vi "Unevenly Sampled Signal Spectrum.vi"(0 "XTime":dbl[](array[numeric]), 1 "X":dbl[](array[numeric])) -> (2 "Power Spectrum FFT {X} Frequency":dbl[](array[numeric]), 3 "Power Spectrum FFT {X}":dbl[](array[numeric]), 4 "error":i32)   [LabVIEW 2024, in "NI_Gmath.lvlib"]
doc: "<p>Calculates the power spectrum of a signal that is unevenly spaced in time.</p>"
uses:
  NI_Gmath.lvlib
  Real Dot Product.vi
  NI_AALBase.lvlib
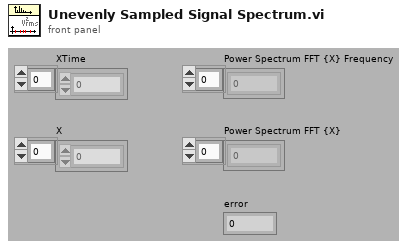
[diagram p1: front panel]
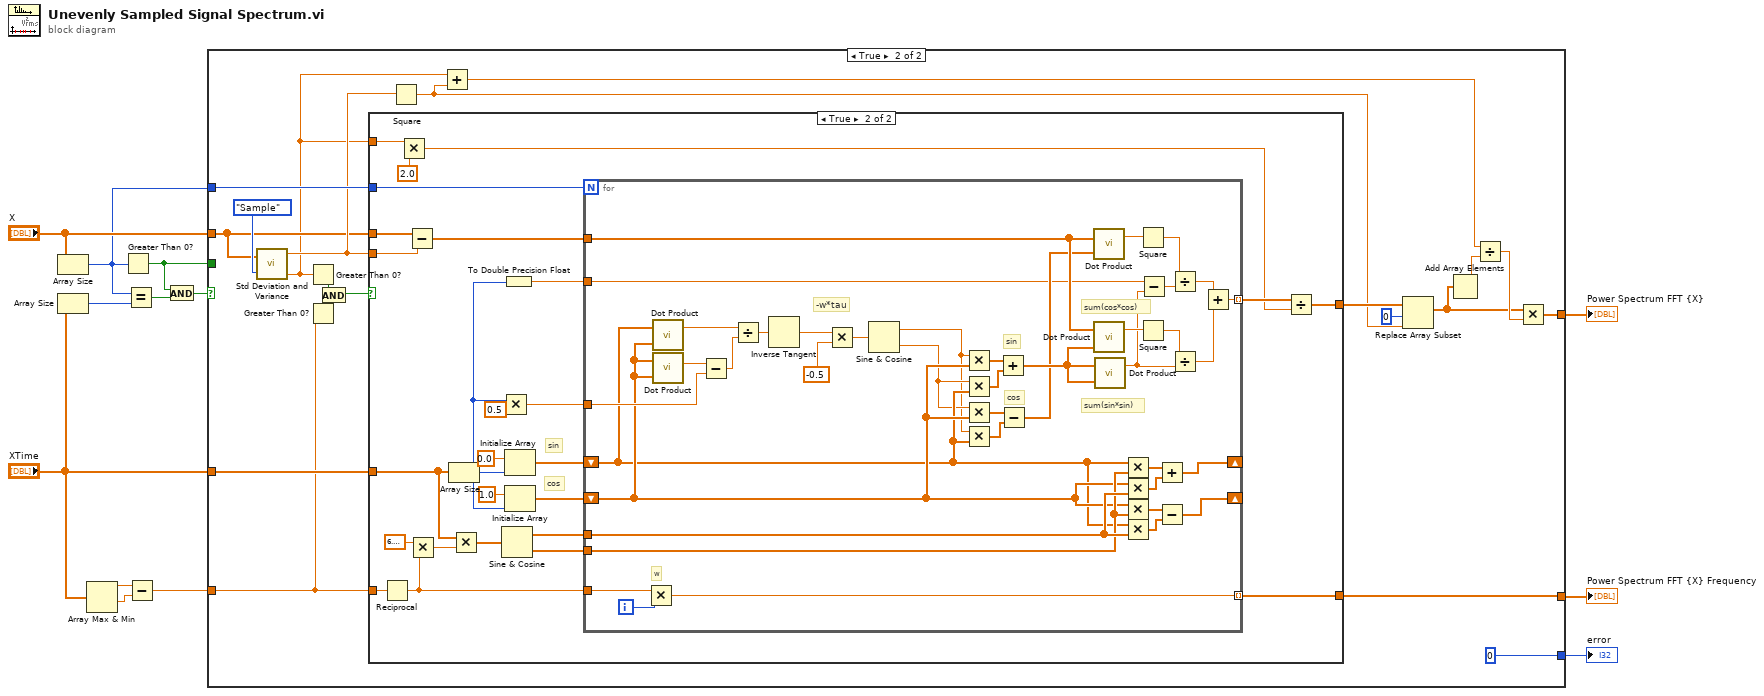
[diagram p0: block diagram]
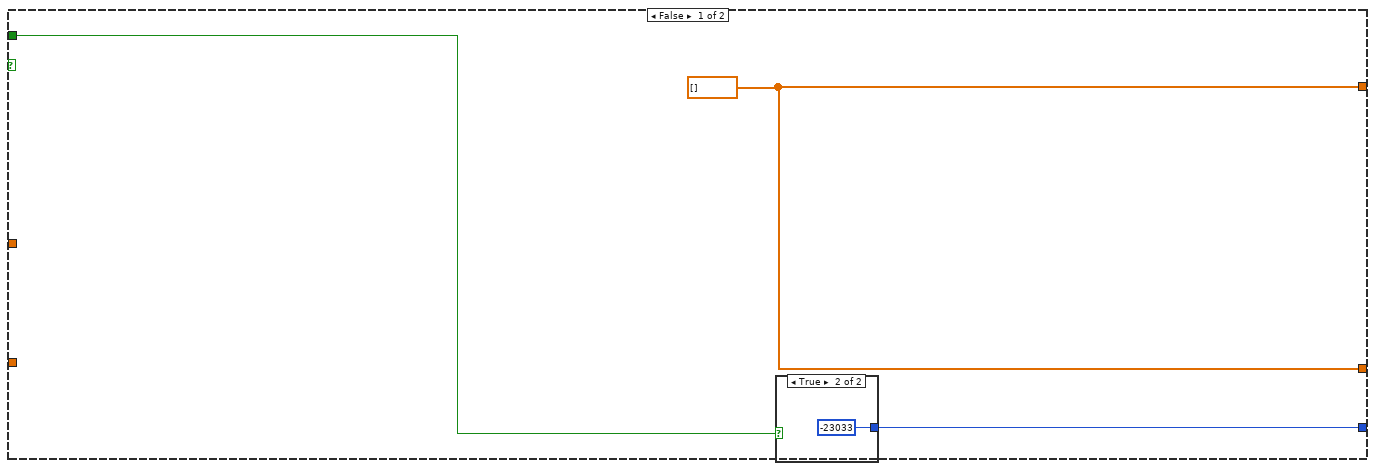
[diagram p2: hidden frame]
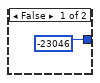
[diagram p3: hidden frame]
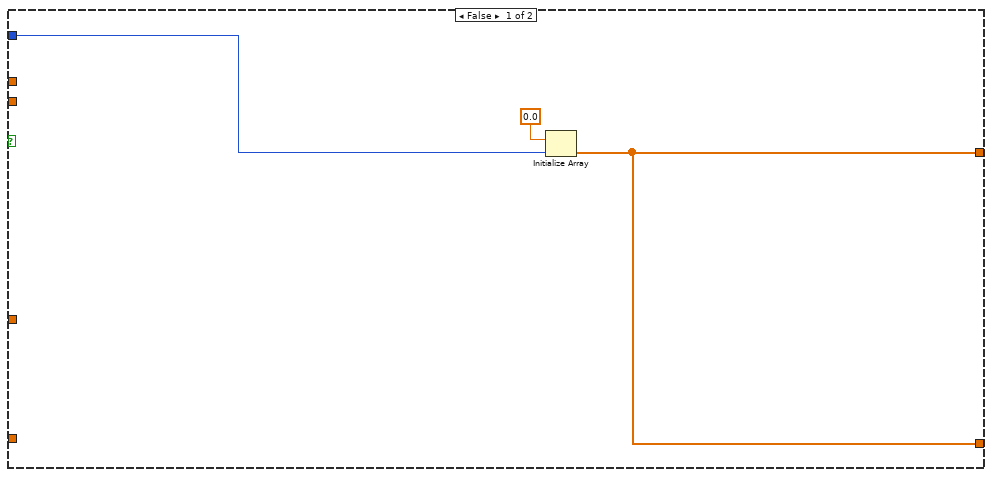
[diagram p4: hidden frame]
diagram:
  n1 = Array Size(array="X") -> (size(s)=w1:i32)
  n2 = Array Size(array="XTime") -> (size(s)=w10:i32)
  n3 = Array Max & Min(array="XTime") -> (max value=w5:dbl, min value=w4:dbl)  [unwired: 2 out]
  n4 = Greater Than 0?(x=w1) -> (x > 0?=w7:bool)
  n5 = Equal?(x=w1, y=w10) -> (x = y?=w9:bool)
  n6 = Subtract(x=w5, y=w4) -> (x-y=w3:dbl)
  n7 = And(x=w7, y=w9) -> (x .and. y?=w8:bool)
  n8 = case shown="True" w8 {
    tunnel: w1 -> [_ w36]
    tunnel: "X" -> [_ w25]
    tunnel: "XTime" -> [_ w38]
    tunnel: [w14 w29] -> w12
    tunnel: [w14 w28] -> w13
    tunnel: [w15 0] -> w11
    tunnel: w7 -> [w16 _]
    tunnel: w3 -> [_ w35]
    frame False {
      w14 = dbl[] []
      n9 = case shown="True" w16 {
        tunnel: [-23046 -23033] -> w15
        frame False {
        }
        frame True {
        }
      }
    }
    frame True {
      n10 = call "Std Deviation and Variance.vi"("X"=w25, "Weighting (Sample)"=enum16{"Sample", "Population"}."Sample") -> ("mean"=w27:dbl, "variance"=w23:dbl)  [unwired: 1 out]
      n11 = Greater Than 0?(x=w23) -> (x > 0?=w34:bool)
      n12 = Greater Than 0?(x=w35) -> (x > 0?=w33:bool)
      n13 = And(x=w34, y=w33) -> (x .and. y?=w32:bool)
      n14 = case shown="True" w32 {
        tunnel: w27 -> [_ w67]
        tunnel: w23 -> [_ w61]
        tunnel: w36 -> [w39 w62]
        tunnel: [w40 w59] -> w31
        tunnel: w38 -> [_ w55]
        tunnel: w25 -> [_ w64]
        tunnel: w35 -> [_ w46]
        tunnel: [w40 w45] -> w28
        frame False {
          n15 = Initialize Array(0.0, w39) -> (w40:dbl[])
        }
        frame True {
          # "cos"
          # "sin"
          n16 = Reciprocal(x=w46) -> (1/x=w44:dbl)
          n17 = Multiply(x=w61, y=2.0) -> (x*y=w58:dbl)
          n18 = Subtract(x=w64, y=w67) -> (x-y=w66:dbl[])
          n19 = Multiply(x=6.283185307179586, y=w44) -> (x*y=w57:dbl)
          n20 = Array Size(array=w55) -> (size(s)=w43:i32)
          n21 = Multiply(x=w55, y=w57) -> (x*y=w56:dbl[])
          n22 = Multiply(x=w43, y=0.5) -> (x*y=w47:dbl)
          n23 = Sine & Cosine(0:w56) -> (1:w51:dbl[], 2:w50:dbl[])
          n24 = To Double Precision Float(number=w43) -> (double precision float=w42:dbl)
          n25 = Initialize Array(0.0 ("element"), w43) -> (w53:dbl[])
          n26 = Initialize Array(1.0 ("element"), w43) -> (w52:dbl[])
          n27 = for {
            N: w62 -> [_]
            tunnel: [w73] -> w45 mode=indexing
            tunnel: w66 -> [w102]
            tunnel: [w96] -> w60 mode=indexing
            tunnel: w44 -> [w97]
            shift-right: [w93] -> _
            shift-left: w53 -> [w78]
            shift-right: [w90] -> _
            shift-left: w52 -> [w79]
            tunnel: w51 -> [w89]
            tunnel: w50 -> [w88]
            tunnel: w47 -> [w85]
            tunnel: w42 -> [w68]
            i -> [w107]
            # "sum(cos*cos)"
            # "sum(sin*sin)"
            # "cos"
            # "sin"
            # "w"
            # "-w*tau"
            n28 = Multiply(x=w97, y=w107) -> (x*y=w73:dbl)
            n29 = call-poly "Dot Product.vi"("Y Vector"=w79, "X Vector"=w78) -> ("X * Y"=w87:dbl)  [unwired: 1 out]
            n30 = call-poly "Dot Product.vi"("Y Vector"=w79, "X Vector"=w79) -> ("X * Y"=w86:dbl)  [unwired: 1 out]
            n31 = Subtract(x=w86, y=w85) -> (x-y=w84:dbl)
            n32 = Divide(x=w87, y=w84) -> (x/y=w106:dbl)
            n33 = Inverse Tangent(1:w106) -> (0:w105:dbl)
            n34 = Multiply(x=w105, y=-0.5) -> (x*y=w72:dbl)
            n35 = Sine & Cosine(0:w72) -> (1:w76:dbl, 2:w77:dbl)
            n36 = Multiply(x=w76, y=w79) -> (x*y=w83:dbl[])
            n37 = Multiply(x=w77, y=w78) -> (x*y=w82:dbl[])
            n38 = Multiply(x=w77, y=w79) -> (x*y=w80:dbl[])
            n39 = Multiply(x=w76, y=w78) -> (x*y=w81:dbl[])
            n40 = Add(x=w83, y=w82) -> (x+y=w75:dbl[])
            n41 = Subtract(x=w80, y=w81) -> (x-y=w74:dbl[])
            n42 = call-poly "Dot Product.vi"("Y Vector"=w74, "X Vector"=w102) -> ("X * Y"=w104:dbl)  [unwired: 1 out]
            n43 = call-poly "Dot Product.vi"("Y Vector"=w75, "X Vector"=w102) -> ("X * Y"=w101:dbl)  [unwired: 1 out]
            n44 = call-poly "Dot Product.vi"("Y Vector"=w75, "X Vector"=w75) -> ("X * Y"=w69:dbl)  [unwired: 1 out]
            n45 = Multiply(x=w78, y=w88) -> (x*y=w95:dbl[])
            n46 = Multiply(x=w79, y=w89) -> (x*y=w94:dbl[])
            n47 = Multiply(x=w79, y=w88) -> (x*y=w92:dbl[])
            n48 = Multiply(x=w78, y=w89) -> (x*y=w91:dbl[])
            n49 = Square(x=w104) -> (x^2=w103:dbl)
            n50 = Square(x=w101) -> (x^2=w100:dbl)
            n51 = Subtract(x=w68, y=w69) -> (x-y=w70:dbl)
            n52 = Add(x=w95, y=w94) -> (x+y=w93:dbl[])
            n53 = Subtract(x=w92, y=w91) -> (x-y=w90:dbl[])
            n54 = Divide(x=w103, y=w70) -> (x/y=w99:dbl)
            n55 = Divide(x=w100, y=w69) -> (x/y=w98:dbl)
            n56 = Add(x=w99, y=w98) -> (x+y=w96:dbl)
          }
          n57 = Divide(x=w60, y=w58) -> (x/y=w59:dbl[])
        }
      }
      n58 = Square(x=w27) -> (x^2=w24:dbl)
      n59 = Add(x=w23, y=w24) -> (x+y=w22:dbl)
      n60 = Replace Array Subset(array=w31, new element=w24, index=0) -> (w19:dbl[])
      n61 = Add Array Elements(numeric array=w19) -> (sum=w21:dbl)
      n62 = Divide(x=w22, y=w21) -> (x/y=w20:dbl)
      n63 = Multiply(x=w19, y=w20) -> (x*y=w29:dbl[])
    }
  }
  "Power Spectrum FFT {X}" <- w12
  "error" <- w11
  "Power Spectrum FFT {X} Frequency" <- w13
